vi "CRC.vi"(8 "error in (no error)":errorcluster, 11 "puchMsg":string) -> (0 "error out":errorcluster, 1 "CRC校验":string, 2 "数据段":string, 3 "数据段长度":string)   [LabVIEW 2016, in "212format_work.lvclass"]
uses:
  212format_work.lvclass
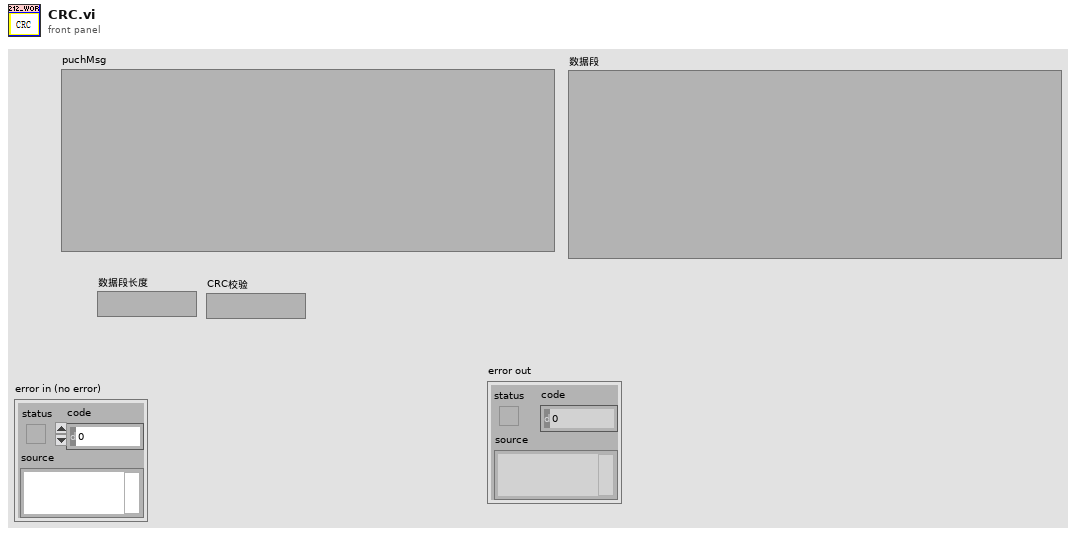
[diagram p1: front panel]
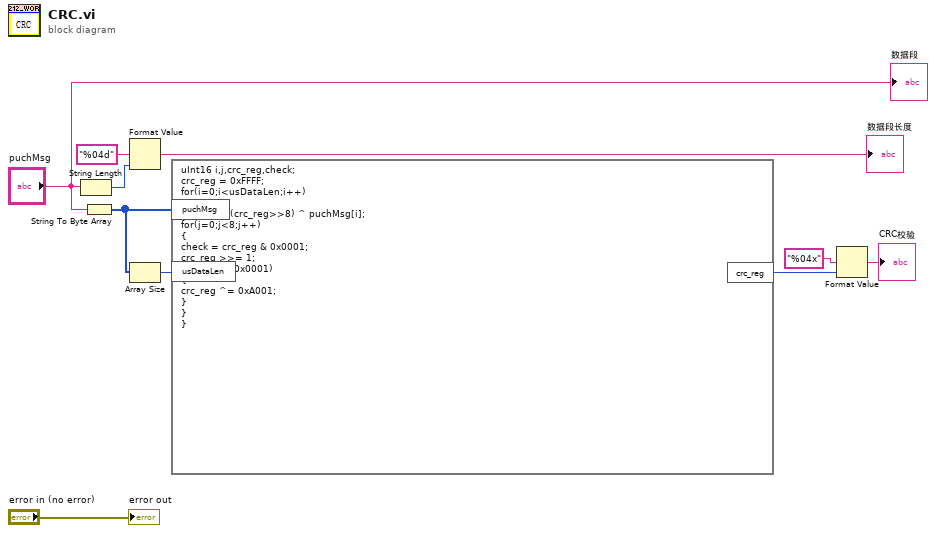
[diagram p0: block diagram]
diagram:
  n1 = String Length(string="puchMsg") -> (length=w8:i32)
  n2 = String To Byte Array(string="puchMsg") -> (unsigned byte array=w10:u8[])
  n3 = Format Value(format string="%04d" ("格式字符串"), value (0)=w8) -> (output string=→"数据段长度":string)  [unwired: 1 in]
  n4 = Array Size(array=w10) -> (size(s)=w9:i32)
  n5 = formula code="uInt16 i,j,crc_reg,check;\ncrc_reg = 0xFFFF;\nfor(i=0;i<usDataLen;i++)\n{\ncrc_reg = (crc_reg>>8) ^ puchMsg[i];\nfor(j=0;j<8;j++)\n{\ncheck = crc_reg & 0x0001;\ncrc_reg >>= 1;\nif(check==0x0001)\n{\ncrc_reg ^= 0xA001;\n}\n}\n}"("puchMsg"=w10, "usDataLen"=w9) -> ("crc_reg"=w3:u16)
  n6 = Format Value(format string="%04x" ("格式字符串"), value (0)=w3) -> (output string=→"CRC校验":string)  [unwired: 1 in]
  "数据段" <- "puchMsg"
  "error out" <- "error in (no error)"
